vi "Set Channel Property.vi"(5 "Value":variant, 7 "Name":string, 8 "error in (no error)":errorcluster, 9 "Channel Name in":string, 10 "Group Name in":string, 11 "TDMS Log File Specification in":refnum<class "TDMS Log File Specification.lvclass">) -> (0 "error out":errorcluster, 1 "Channel Name out":string, 2 "Group Name out":string, 3 "TDMS Log File Specification out":refnum<class "TDMS Log File Specification.lvclass">)   [LabVIEW 2015, in "Waveform Data Logger Shared.lvlib" / "TDMS Log File Specification.lvclass"]
uses:
  TDMS Log File Specification.lvclass
  TDMS Log File Specification.lvclass/TDMS Log File Specification.ctl
  Property Specification.ctl
  Channel Specification.ctl
  Channel Group Specification.ctl
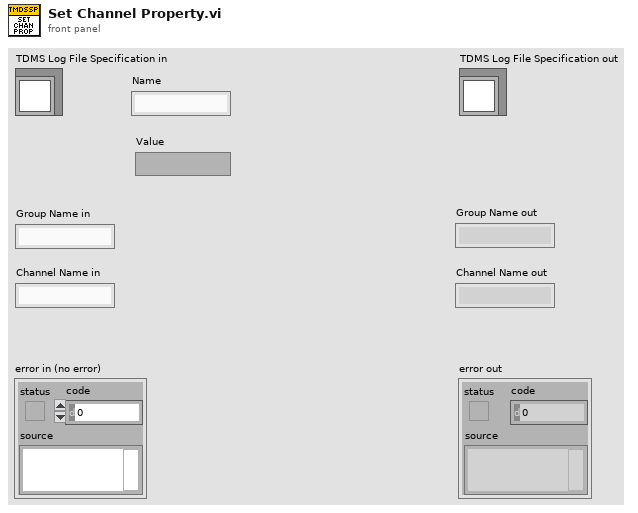
[diagram p1: front panel]
types:
  T1 = typedef "Waveform Data Logger Shared.lvlib/TDMS Log File Specification.lvclass/Property Specification.ctl" = cluster{"Name":string, "Value":variant}
  T2 = typedef "Waveform Data Logger Shared.lvlib/TDMS Log File Specification.lvclass/Channel Specification.ctl" = cluster{"Name":string, "Properties":T1[]}
  T3 = typedef "Waveform Data Logger Shared.lvlib/TDMS Log File Specification.lvclass/Channel Group Specification.ctl" = cluster{"Name":string, "Properties":T1[], "Channels":T2[]}
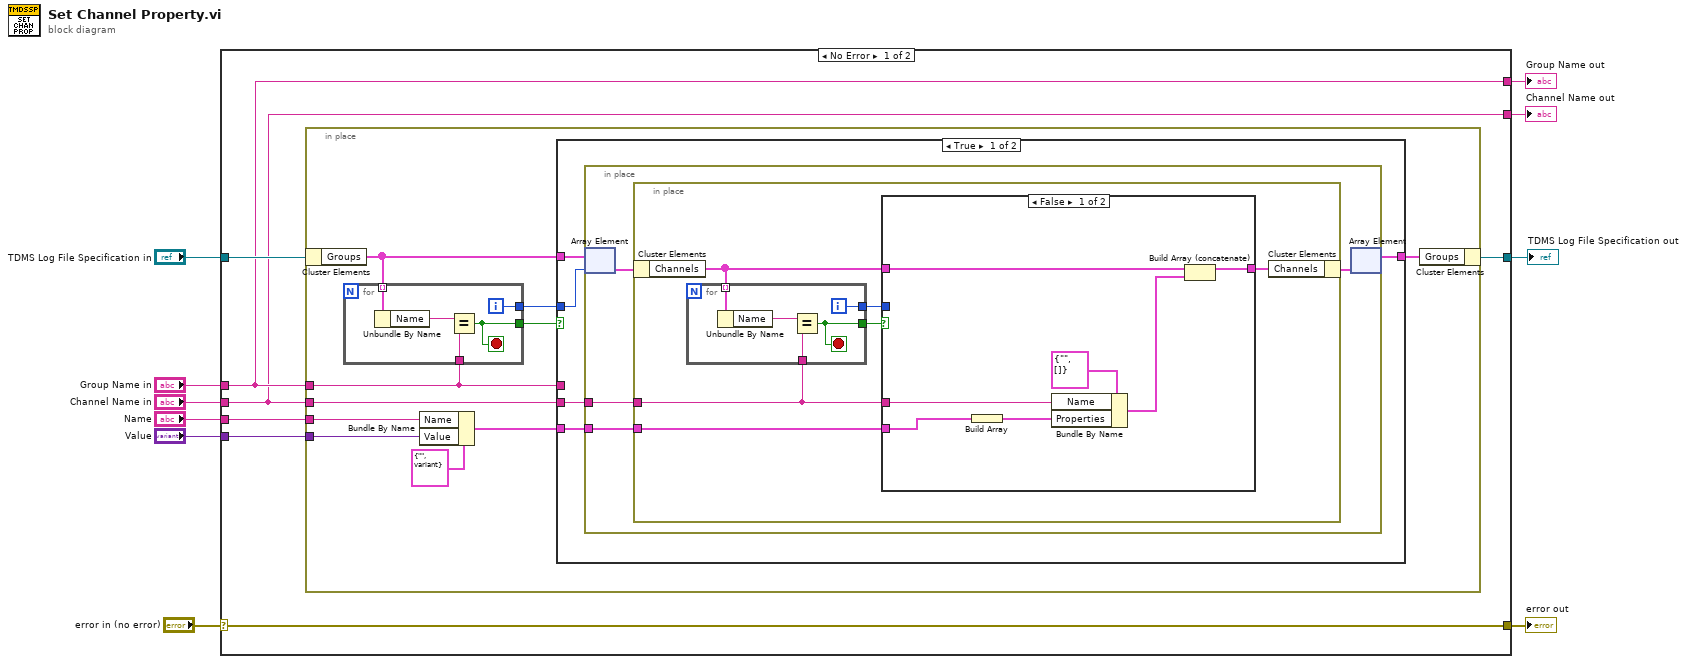
[diagram p0: block diagram]
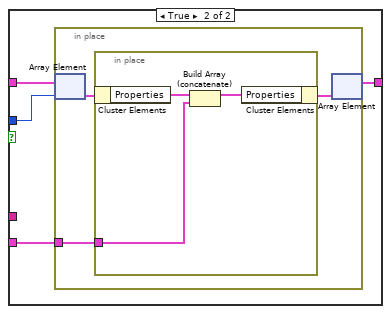
[diagram p2: hidden frame]
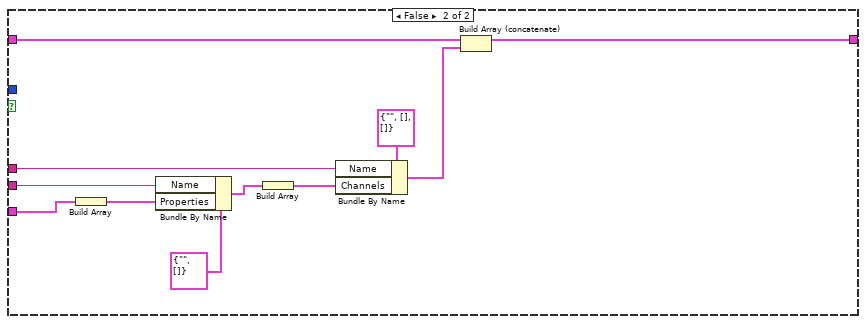
[diagram p3: hidden frame]
diagram:
  n1 = case shown="No Error" "error in (no error)" {
    selector: "error in (no error)" -> [w17 w84]
    tunnel: [w17 w84] -> w8
    tunnel: [w13 w83] -> w6
    tunnel: "TDMS Log File Specification in" -> [w16 w83]
    tunnel: "Name" -> [w15 _]
    tunnel: "Value" -> [w14 _]
    tunnel: "Group Name in" -> [w12 w82]
    tunnel: "Channel Name in" -> [w11 w81]
    tunnel: [w12 w82] -> w2
    tunnel: [w11 w81] -> w1
    frame No Error {
      n2 = in-place {
        in-place-border: w15 -> [w26]
        in-place-border: w14 -> [w25]
        in-place-border: w12 -> [w19]
        in-place-border: w11 -> [w18]
        n3 = in-place-cluster #1(w16) -> ("Groups"=w22:T3[])
        n4 = for {
          tunnel: w22 -> [w80] mode=indexing
          tunnel: w19 -> [w78]
          tunnel: [w77] -> w24
          tunnel: [w76] -> w23
          i -> [w76]
          stop <- w77 stop-if-true
          n5 = Unbundle By Name(w80) -> ("Name"=w79:string)
          n6 = Equal?(x=w79, y=w78) -> (x = y?=w77:bool)
        }
        n7 = Bundle By Name(cluster=T1 {"Name"="", "Value"=variant} ("Property"), "Name"=w26, "Value"=w25) -> (w21:T1)
        n8 = case shown="True" w24 {
          tunnel: w23 -> [w31 _]
          tunnel: w22 -> [w32 w75]
          tunnel: w21 -> [w30 w66]
          tunnel: [w29 w74] -> w20
          tunnel: w19 -> [_ w72]
          tunnel: w18 -> [w28 w69]
          frame True {
            n9 = in-place {
              in-place-border: w30 -> [w35]
              in-place-border: w28 -> [w33]
              n10 = in-place-array #2(w32, w31) -> (w36:T3)
              n11 = in-place {
                in-place-border: w35 -> [w39]
                in-place-border: w33 -> [w38]
                n12 = in-place-cluster #3(w36) -> ("Channels"=w40:T2[])
                n13 = for {
                  tunnel: w40 -> [w64] mode=indexing
                  tunnel: w38 -> [w62]
                  tunnel: [w61] -> w42
                  tunnel: [w60] -> w41
                  i -> [w60]
                  stop <- w61 stop-if-true
                  n14 = Unbundle By Name(w64) -> ("Name"=w63:string)
                  n15 = Equal?(x=w63, y=w62) -> (x = y?=w61:bool)
                }
                n16 = case shown="False" w42 {
                  tunnel: w41 -> [_ w51]
                  tunnel: w40 -> [w45 w53]
                  tunnel: w39 -> [w46 w52]
                  tunnel: w38 -> [w47 _]
                  tunnel: [w43 w50] -> w37
                  frame False {
                    n17 = Build Array(w46) -> (w48:T1[])
                    n18 = Bundle By Name(cluster=T2 {"Name"="", "Properties"=[]} ("Channel Specification"), "Name"=w47, "Properties"=w48) -> (w44:T2)
                    n19 = Build Array (concatenate)(w45, w44) -> (w43:T2[])
                  }
                  frame True {
                    n20 = in-place {
                      in-place-border: w52 -> [w54]
                      n21 = in-place-array #4(w53, w51) -> (w56:T2)
                      n22 = in-place {
                        in-place-border: w54 -> [w57]
                        n23 = in-place-cluster #5(w56) -> ("Properties"=w59:T1[])
                        n24 = Build Array (concatenate)(w59, w57) -> (w58:T1[])
                        n25 = in-place-cluster #5("Properties"=w58) -> (w55:T2)
                      }
                      n26 = in-place-array #4(w55) -> (w50:T2[])  [unwired: 1 out]
                    }
                  }
                }
                n27 = in-place-cluster #3("Channels"=w37) -> (w34:T3)
              }
              n28 = in-place-array #2(w34) -> (w29:T3[])  [unwired: 1 out]
            }
          }
          frame False {
            n29 = Build Array(w66) -> (w65:T1[])
            n30 = Bundle By Name(cluster=T2 {"Name"="", "Properties"=[]} ("Channel Specification"), "Name"=w69, "Properties"=w65) -> (w68:T2)
            n31 = Build Array(w68) -> (w67:T2[])
            n32 = Bundle By Name(cluster=T3 {"Name"="", "Properties"=[], "Channels"=[]} ("Group Specification"), "Name"=w72, "Channels"=w67) -> (w71:T3)
            n33 = Build Array (concatenate)(w75, w71) -> (w74:T3[])
          }
        }
        n34 = in-place-cluster #1("Groups"=w20) -> (w13:refnum<class "TDMS Log File Specification.lvclass">)
      }
    }
    frame Error {
    }
  }
  "error out" <- w8
  "TDMS Log File Specification out" <- w6
  "Group Name out" <- w2
  "Channel Name out" <- w1
